vi "Device under test (subVI).vi"(8 "error in (no error)":errorcluster, 11 "signal in":waveform(dbl)) -> (0 "error out":errorcluster, 3 "stimulus and response":waveform(dbl)[](array[waveform]))   [LabVIEW 2020]
doc: "Uses a Lowpass Elliptic filter (8th order)."
uses:
  <vilib>/measure/macond.llb/IIR Filter for 1 Chan.vi
  <vilib>/measure/NI_MAPro.lvlib
panel:
  # "OUTPUT = array containing two waveforms\nWaveform 0: Stimulus\nWaveform 1: Response"
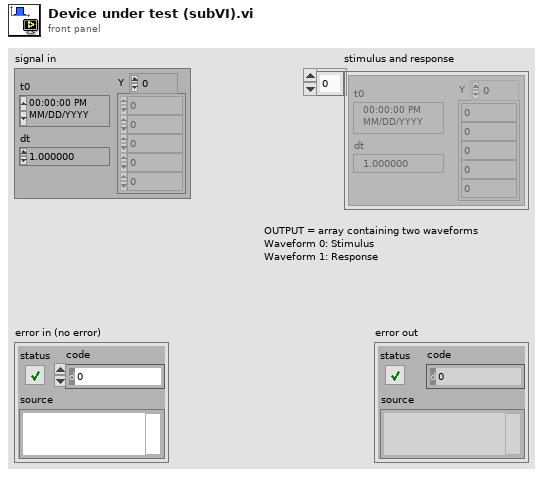
[diagram p1: front panel]
types:
  T1 = cluster{"Topology":enum16{"Off", "Butterworth", "Chebyshev", "Inverse Chebyshev", "Elliptic", "Bessel"}, "Type":enum16{"Lowpass", "Highpass", "Bandpass", "Bandstop"}, "Order":i32, "Lower Fc":dbl, "Upper Fc":dbl, "PB Ripple":dbl, "SB Attenuation":dbl}
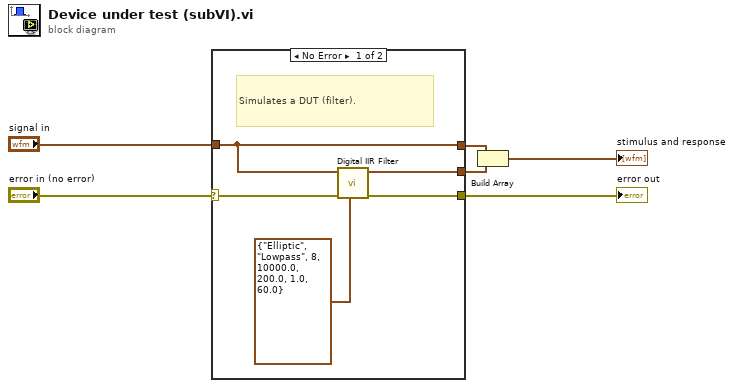
[diagram p0: block diagram]
diagram:
  n1 = case shown="No Error" "error in (no error)" {
    selector: "error in (no error)" -> [w7 w13]
    tunnel: [w11 w13] -> w5
    tunnel: "signal in" -> [w9 w12]
    tunnel: [w10 w12] -> w3
    tunnel: [w9 w12] -> w2
    frame No Error {
      # "Simulates a DUT (filter)."
      # "Simulates a DUT(filter)"
      n2 = call-poly <vilib>:"Digital IIR Filter.vi"("IIR filter specifications"=T1 {"Topology"=enum."Elliptic", "Type"=enum."Lowpass", "Order"=8, "Lower Fc"=10000.0, "Upper Fc"=200.0, "PB Ripple"=1.0, "SB Attenuation"=60.0}, "error in (no error)"=w7, "signal in"=w9) -> ("error out"=w11:errorcluster, "signal out"=w10:waveform(dbl))  [unwired: 6 in, 1 out]
    }
    frame Error {
    }
  }
  "error out" <- w5
  n3 = Build Array(w2, w3) -> (→"stimulus and response":waveform(dbl)[])
